vi "Exit_All_Loops.vi"(8 "error in (no error)":errorcluster, 9 "10Hz_Q":refnum<queue>, 10 "Noise_Q":refnum<queue>, 11 "Tones_Q":refnum<queue>) -> (0 "error out":errorcluster)   [LabVIEW 2018]
uses:
  Controls/Enums/NoiseQueueElements.ctl
  Queue/DataQueueElements.ctl
  Controls/Enums/10Hz_Loop_Enum.ctl
  Controls/Enums/DigiLoopEnum.ctl
  Controls/Enums/LogLoopEnum.ctl
  Controls/Enums/FP_Loop_Enum.ctl
  Controls/Enums/PXI_Loop_Enum.ctl
  NASA/statmon_2015/health_state.ctl
  Controls/Enums/AO_Loop_Enum.ctl
  Controls/Enums/UPS_Loop_Enum.ctl
  Controls/Enums/TCP_Loop.ctl
  Controls/Enums/AI_Loop_Enum.ctl
  Queue/HWQueueElements.ctl
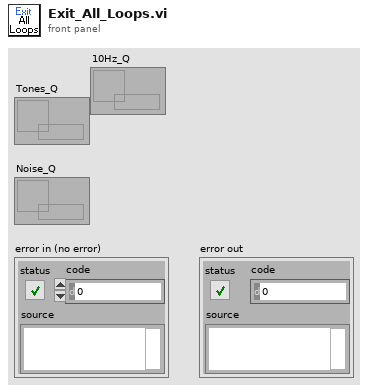
[diagram p1: front panel]
types:
  T1 = typedef "TCP_Loop.ctl" = enum16{"TCP_Write", "TCP_ChkTime", "TCP_Exit"}
  T2 = typedef "10Hz_Loop_Enum.ctl" = enum16{"10Hz_Init", "10Hz_Cfg", "10Hz_NewData", "10Hz_Write", "10Hz_Stop"}
  T3 = typedef "UPS_Loop_Enum.ctl" = enum16{"UPS_Init", "UPS_Read", "UPS_ChkTime", "UPS_Exit"}
  T4 = typedef "AO_Loop_Enum.ctl" = enum16{"AO_Init", "AO_Write", "AO_Exit"}
  T5 = typedef "health_state.ctl" = enum16{"Health_Config", "Health_Wait", "Health_Read", "Health_Log", "Health_Exit"}
  T6 = typedef "PXI_Loop_Enum.ctl" = enum16{"PXI_Init", "PXI_Time", "PXI_Read", "PXI_Exit"}
  T7 = typedef "FP_Loop_Enum.ctl" = enum16{"FP_Init", "FP_Scale", "FP_Tone", "FP_Noise", "FP_Probes", "FP_PXI", "FP_AI", "FP_TC", "FP_PWR_Hist", "FP_Alarm", "FP_Exit"}
  T8 = typedef "LogLoopEnum.ctl" = enum16{"Log_Init", "Log_Config", "Log_CfgAlarm", "Log_TimeDomain", "Log_Tone", "Log_NoiseTrace", "Log_NoiseSum", "Log_DO", "Log_AI", "Log_TC", "Log_Disdrom", "Log_Weather", "Log_TE", "Log_ADAM", "Log_UPS", "Log_ChkTime", "Log_Alarm", "Log_SSH", "Log_Write", "Log_Exit"}
  T9 = typedef "DigiLoopEnum.ctl" = enum16{"Dig_Init", "Digi_Write", "Digi_Exit"}
  T10 = typedef "NoiseQueueElements.ctl" = enum16{"Noise_Startup", "Noise_Init", "Noise_Macro", "Noise_Config", "Noise_NewData", "Noise_Transform", "Noise_SumdTrace", "Noise_Send", "Noise_Probes", "Noise_Exit"}
  T11 = typedef "DataQueueElements.ctl" = enum16{"Data_Init", "Data_Config", "Data_AddData", "Data_FreqShift", "Data_FPGA_Write", "Data_Transform", "Data_Send", "Data_Exit"}
  T12 = typedef "HWQueueElements.ctl" = enum16{"HW_Init", "HW_UpdtCfg", "HW_Start", "HW_Pause", "HW_Run", "HW_Cls", "HW_Exit"}
  T13 = typedef "AI_Loop_Enum.ctl" = enum16{"AI_Init", "AI_Config", "AI_Alarm", "AI_Read", "AI_ChkTime", "AI_Exit"}
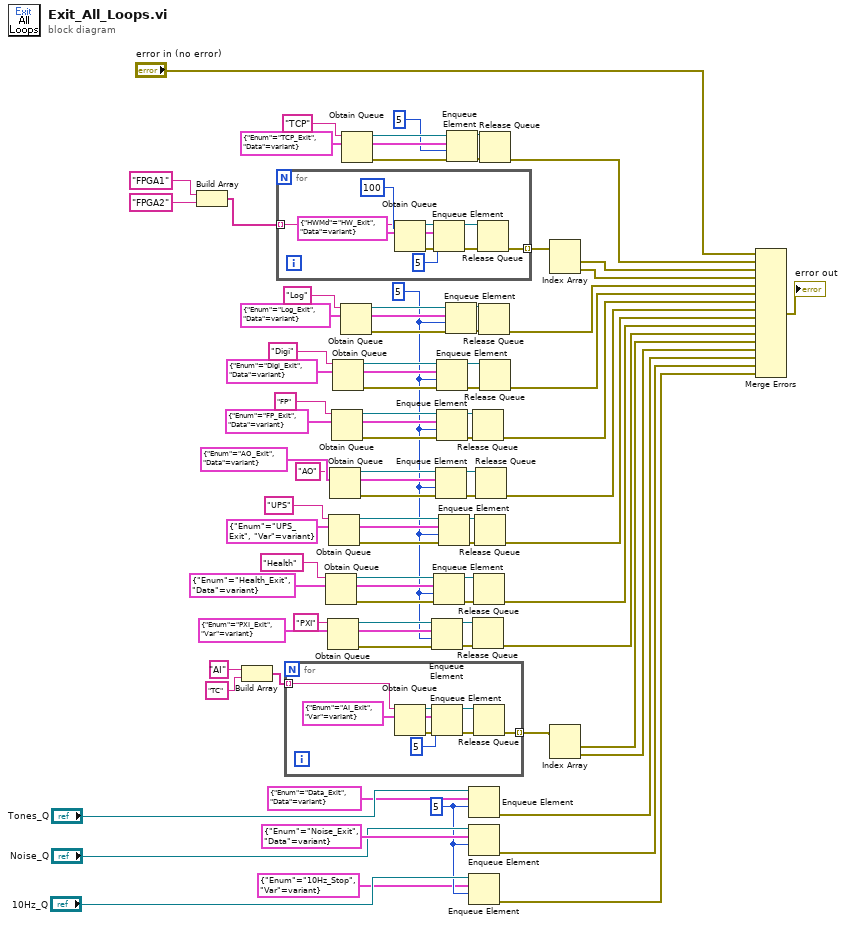
[diagram p0: block diagram]
diagram:
  w6 = cluster{"Enum":T1, "Data":variant} {"Enum"=enum."TCP_Exit", "Data"=variant}
  w10 = 5 ("timeout in ms (-1)")
  w13 = 5 ("timeout in ms (-1)")
  w31 = cluster{"Enum":T3, "Var":variant} {"Enum"=enum."UPS_Exit", "Var"=variant}
  w76 = cluster{"Enum":T4, "Data":variant} {"Enum"=enum."AO_Exit", "Data"=variant}
  w69 = cluster{"Enum":T5, "Data":variant} {"Enum"=enum."Health_Exit", "Data"=variant}
  w63 = cluster{"Enum":T6, "Var":variant} {"Enum"=enum."PXI_Exit", "Var"=variant}
  w56 = cluster{"Enum":T7, "Data":variant} {"Enum"=enum."FP_Exit", "Data"=variant}
  w54 = cluster{"Enum":T8, "Data":variant} {"Enum"=enum."Log_Exit", "Data"=variant}
  w49 = cluster{"Enum":T9, "Data":variant} {"Enum"=enum."Digi_Exit", "Data"=variant}
  n1 = Build Array("FPGA1" ("name (unnamed)"), "FPGA2" ("name (unnamed)")) -> (w60:string[])
  n2 = Build Array("AI" ("name (unnamed)"), "TC" ("name (unnamed)")) -> (w71:string[])
  n3 = for {
    tunnel: w60 -> [w87] mode=indexing
    tunnel: [w85] -> w30 mode=indexing
    w88 = cluster{"HWMd":T12, "Data":variant} {"HWMd"=enum."HW_Exit", "Data"=variant}
    n4 = Obtain Queue(max queue size (-1, unlimited)=100, name (unnamed)=w87, element data type=w88) -> (queue out=w89:refnum<queue>, error out=w90:errorcluster)  [unwired: 2 in, 1 out]
    n5 = Enqueue Element(queue=w89, element=w88, timeout in ms (-1)=5, error in (no error)=w90) -> (queue out=w84:refnum<queue>, error out=w86:errorcluster)  [unwired: 1 out]
    n6 = Release Queue(queue=w84, error in (no error)=w86) -> (error out=w85:errorcluster)  [unwired: 1 in, 2 out]
  }
  n7 = for {
    tunnel: w71 -> [w98] mode=indexing
    tunnel: [w94] -> w16 mode=indexing
    w96 = cluster{"Enum":T13, "Var":variant} {"Enum"=enum."AI_Exit", "Var"=variant}
    n8 = Obtain Queue(name (unnamed)=w98, element data type=w96) -> (queue out=w99:refnum<queue>, error out=w97:errorcluster)  [unwired: 3 in, 1 out]
    n9 = Enqueue Element(queue=w99, element=w96, timeout in ms (-1)=5, error in (no error)=w97) -> (queue out=w93:refnum<queue>, error out=w95:errorcluster)  [unwired: 1 out]
    n10 = Release Queue(queue=w93, error in (no error)=w95) -> (error out=w94:errorcluster)  [unwired: 1 in, 2 out]
  }
  n11 = Obtain Queue(name (unnamed)="Health", element data type=w69) -> (queue out=w67:refnum<queue>, error out=w68:errorcluster)  [unwired: 3 in, 1 out]
  n12 = Obtain Queue(name (unnamed)="PXI", element data type=w63) -> (queue out=w62:refnum<queue>, error out=w65:errorcluster)  [unwired: 3 in, 1 out]
  n13 = Obtain Queue(name (unnamed)="UPS", element data type=w31) -> (queue out=w32:refnum<queue>, error out=w34:errorcluster)  [unwired: 3 in, 1 out]
  n14 = Obtain Queue(name (unnamed)="AO", element data type=w76) -> (queue out=w73:refnum<queue>, error out=w74:errorcluster)  [unwired: 3 in, 1 out]
  n15 = Obtain Queue(name (unnamed)="FP", element data type=w56) -> (queue out=w57:refnum<queue>, error out=w58:errorcluster)  [unwired: 3 in, 1 out]
  n16 = Obtain Queue(name (unnamed)="Digi", element data type=w49) -> (queue out=w50:refnum<queue>, error out=w48:errorcluster)  [unwired: 3 in, 1 out]
  n17 = Obtain Queue(name (unnamed)="Log", element data type=w54) -> (queue out=w53:refnum<queue>, error out=w52:errorcluster)  [unwired: 3 in, 1 out]
  n18 = Obtain Queue(name (unnamed)="TCP", element data type=w6) -> (queue out=w5:refnum<queue>, error out=w4:errorcluster)  [unwired: 3 in, 1 out]
  n19 = Enqueue Element(queue=w62, element=w63, timeout in ms (-1)=w13, error in (no error)=w65) -> (queue out=w37:refnum<queue>, error out=w38:errorcluster)  [unwired: 1 out]
  n20 = Enqueue Element(queue=w67, element=w69, timeout in ms (-1)=w13, error in (no error)=w68) -> (queue out=w39:refnum<queue>, error out=w40:errorcluster)  [unwired: 1 out]
  n21 = Enqueue Element(queue=w73, element=w76, timeout in ms (-1)=w13, error in (no error)=w74) -> (queue out=w77:refnum<queue>, error out=w78:errorcluster)  [unwired: 1 out]
  n22 = Enqueue Element(queue=w50, element=w49, timeout in ms (-1)=w13, error in (no error)=w48) -> (queue out=w41:refnum<queue>, error out=w42:errorcluster)  [unwired: 1 out]
  n23 = Enqueue Element(queue=w57, element=w56, timeout in ms (-1)=w13, error in (no error)=w58) -> (queue out=w80:refnum<queue>, error out=w79:errorcluster)  [unwired: 1 out]
  n24 = Enqueue Element(queue=w32, element=w31, timeout in ms (-1)=w13, error in (no error)=w34) -> (queue out=w35:refnum<queue>, error out=w33:errorcluster)  [unwired: 1 out]
  n25 = Enqueue Element(queue=w53, element=w54, timeout in ms (-1)=w13, error in (no error)=w52) -> (queue out=w82:refnum<queue>, error out=w81:errorcluster)  [unwired: 1 out]
  n26 = Enqueue Element(queue=w5, element=w6, timeout in ms (-1)=5, error in (no error)=w4) -> (queue out=w8:refnum<queue>, error out=w7:errorcluster)  [unwired: 1 out]
  n27 = Enqueue Element(queue="Tones_Q", element=cluster{"Enum":T11, "Data":variant} {"Enum"=enum."Data_Exit", "Data"=variant}, timeout in ms (-1)=w10) -> (error out=w19:errorcluster)  [unwired: 1 in, 2 out]
  n28 = Enqueue Element(queue="Noise_Q", element=cluster{"Enum":T10, "Data":variant} {"Enum"=enum."Noise_Exit", "Data"=variant}, timeout in ms (-1)=w10) -> (error out=w18:errorcluster)  [unwired: 1 in, 2 out]
  n29 = Enqueue Element(queue="10Hz_Q", element=cluster{"Enum":T2, "Var":variant} {"Enum"=enum."10Hz_Stop", "Var"=variant}, timeout in ms (-1)=w10) -> (error out=w11:errorcluster)  [unwired: 1 in, 2 out]
  n30 = Release Queue(queue=w80, error in (no error)=w79) -> (error out=w26:errorcluster)  [unwired: 1 in, 2 out]
  n31 = Release Queue(queue=w37, error in (no error)=w38) -> (error out=w20:errorcluster)  [unwired: 1 in, 2 out]
  n32 = Release Queue(queue=w39, error in (no error)=w40) -> (error out=w21:errorcluster)  [unwired: 1 in, 2 out]
  n33 = Release Queue(queue=w35, error in (no error)=w33) -> (error out=w24:errorcluster)  [unwired: 1 in, 2 out]
  n34 = Release Queue(queue=w77, error in (no error)=w78) -> (error out=w25:errorcluster)  [unwired: 1 in, 2 out]
  n35 = Release Queue(queue=w82, error in (no error)=w81) -> (error out=w28:errorcluster)  [unwired: 1 in, 2 out]
  n36 = Release Queue(queue=w8, error in (no error)=w7) -> (error out=w1:errorcluster)  [unwired: 1 in, 2 out]
  n37 = Release Queue(queue=w41, error in (no error)=w42) -> (error out=w27:errorcluster)  [unwired: 1 in, 2 out]
  n38 = Index Array(array=w30) -> (element #1=w29:errorcluster, element #2=w14:errorcluster)  [unwired: 2 in]
  n39 = Index Array(array=w16) -> (element #1=w17:errorcluster, element #2=w15:errorcluster)  [unwired: 2 in]
  n40 = Merge Errors("error in (no error)", w1, w29, w14, w28, w27, w26, w25, w24, w21, w20, w17, w15, w19, w18, w11) -> (→"error out":errorcluster)
